vi "Import.vi"(8 "error in":errorcluster, 11 "Objects in":T1) -> (0 "error out":errorcluster, 1 "Update":bool, 3 "Objects out":T1)   [LabVIEW 2015, in "tag select module editor node.lvclass"]
uses:
  tag select module editor node.lvclass
  <vilib>/NI/DCAF/Tag Editor Core/Table API/Table Manager/object ref.ctl
  <vilib>/NI/DCAF/Tag Editor Core/Configuration Editor/Classes/Engine Parent/Engine Parent Editor Node.lvclass
  <vilib>/NI/DCAF/Tag Editor Core/Configuration Editor/Classes/Module editor node/module editor node.lvclass
  <vilib>/NI/DCAF/Tag Editor Core/Configuration Editor/Classes/Engine Parent/read engine configuration.vi
  <vilib>/NI/DCAF/Tag Editor Core/Configuration Editor/Classes/Engine Parent/write engine configuration.vi
  <vilib>/NI/Module Execution Interface/Engine Configuration/engine configuration.lvclass
  <vilib>/NI/DCAF/Tag Editor Core/Table API/Table Manager/Table Manager.lvclass
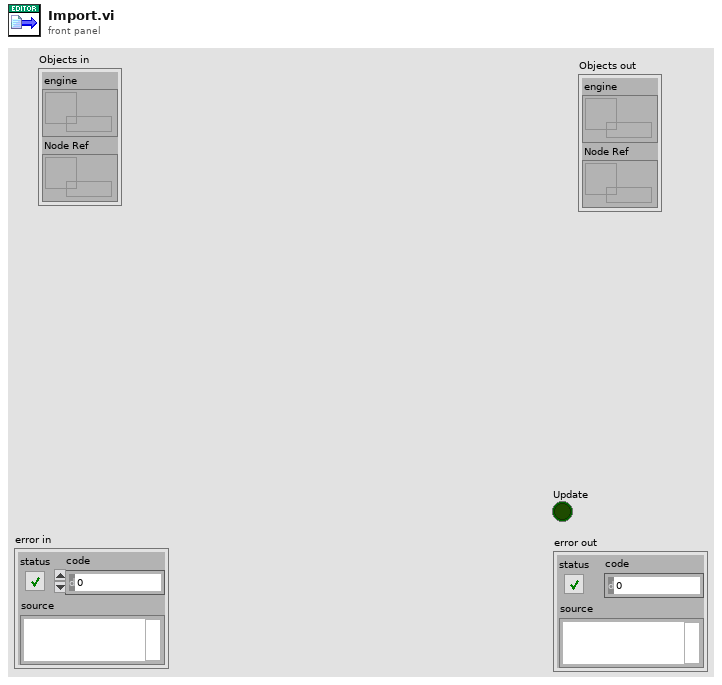
[diagram p1: front panel]
types:
  T1 = typedef "Table Manager.lvlib/Table Manager.lvclass/object ref.ctl" = cluster{"engine":refnum<data-value>, "Node Ref":refnum<data-value>}
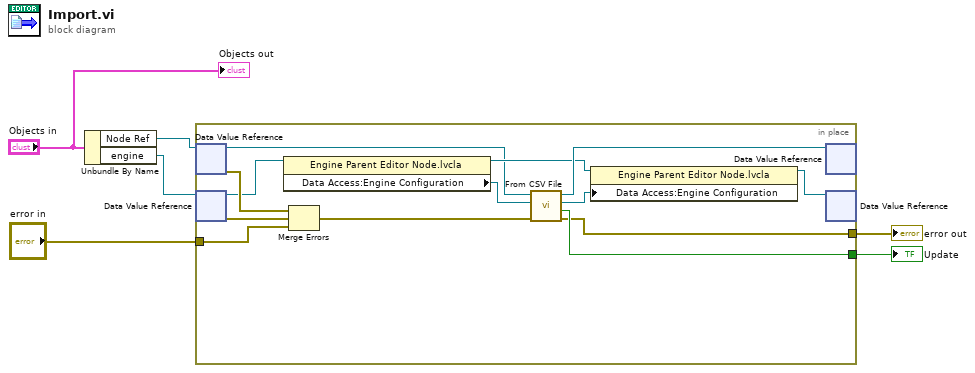
[diagram p0: block diagram]
diagram:
  n1 = Unbundle By Name("Objects in") -> ("Node Ref"=w3:refnum<data-value>, "engine"=w2:refnum<data-value>)
  n2 = in-place {
    in-place-border: "error in" -> [w17]
    in-place-border: [w15] -> w5
    in-place-border: [w14] -> w4
    n3 = in-place-dvr #1(w3) -> (w7:refnum<class "module editor node.lvclass">, w19:errorcluster)
    n4 = in-place-dvr #2(w2) -> (w12:refnum<class "Engine Parent Editor Node.lvclass">, w18:errorcluster)
    n5 = property class="Engine Parent Editor Node.lvcla"(reference=w12) -> (reference out=w9:refnum<class "Engine Parent Editor Node.lvclass">, "Data Access:Engine Configuration"=w11:refnum<class "engine configuration.lvclass">)  [unwired: 1 in, 1 out]
    n6 = Merge Errors(w19, w18, w17) -> (w16:errorcluster)
    n7 = call-dynamic "From CSV File.vi"("error in (no error)"=w16, "engine in"=w11, "module editor node in"=w7) -> ("error out"=w14:errorcluster, "Update"=w15:bool, "engine out"=w10:refnum<class "engine configuration.lvclass">, "module editor node out"=w13:refnum<class "module editor node.lvclass">)  [unwired: 5 in]
    n8 = property class="Engine Parent Editor Node.lvcla"(reference=w9, "Data Access:Engine Configuration"=w10) -> (reference out=w8:refnum<class "Engine Parent Editor Node.lvclass">)  [unwired: 1 in, 1 out]
    n9 = in-place-dvr #1(w13) -> ()  [unwired: 2 out]
    n10 = in-place-dvr #2(w8) -> ()  [unwired: 2 out]
  }
  "error out" <- w4
  "Update" <- w5
  "Objects out" <- "Objects in"
